vi "Get Sibling Classes of Actor.vi"(7 "Target":refnum<vi>, 8 "error in (no error)":errorcluster, 11 "Actor":refnum<vi>) -> (0 "error out":errorcluster, 1 "Sibling Classes":refnum<vi>[](array[refnum]))   [LabVIEW 2020, in "Message Maker.lvlib"]
uses:
  Message Maker.lvlib
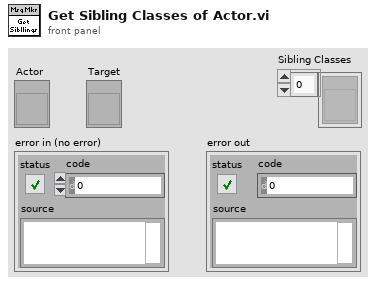
[diagram p1: front panel]
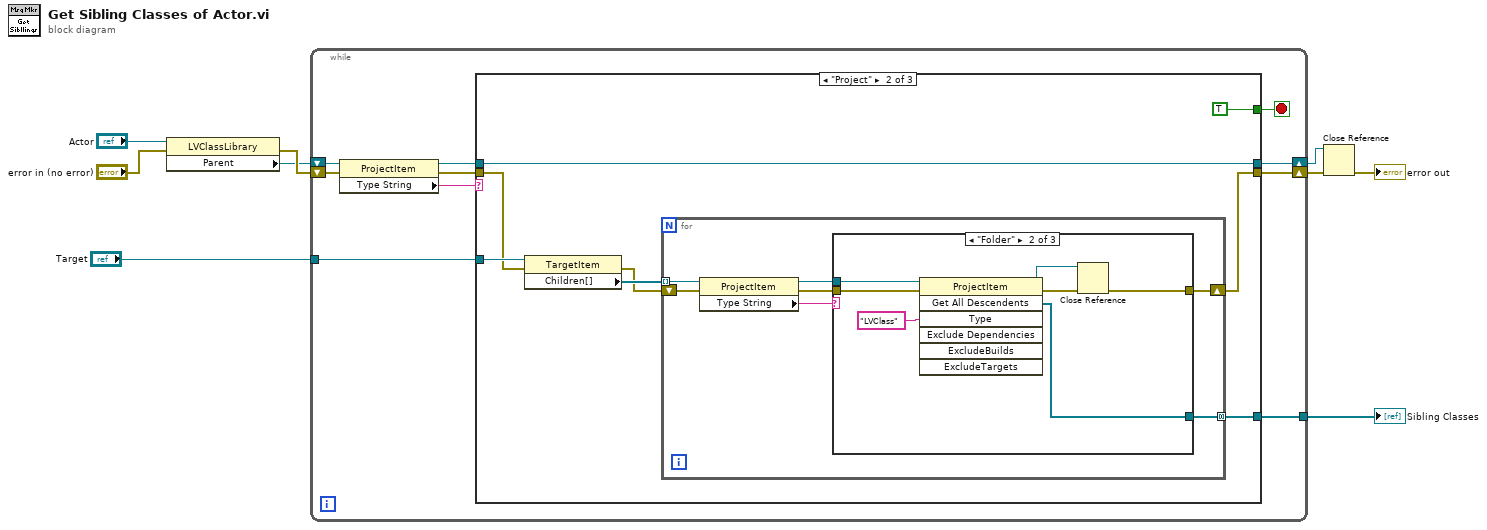
[diagram p0: block diagram]
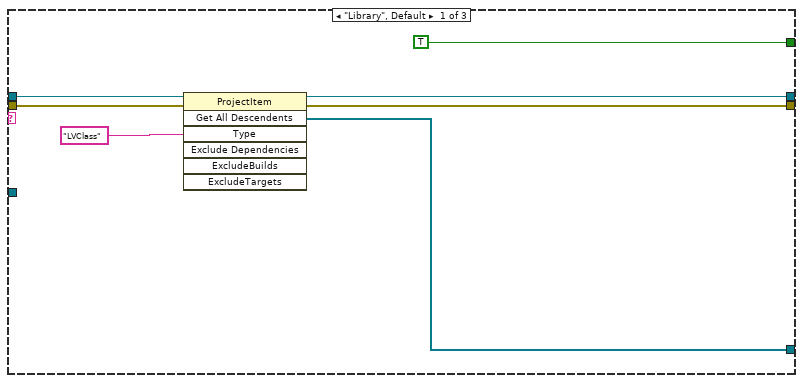
[diagram p2: hidden frame]
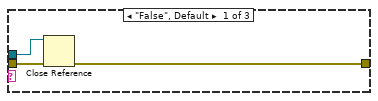
[diagram p3: hidden frame]
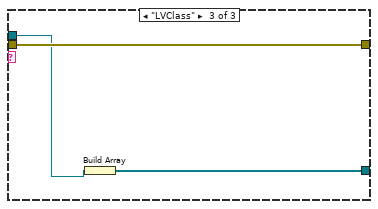
[diagram p4: hidden frame]
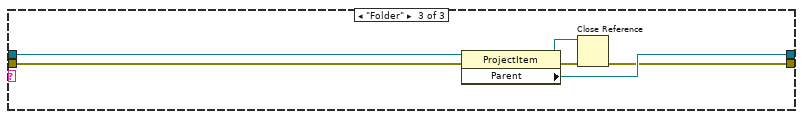
[diagram p5: hidden frame]
diagram:
  n1 = property class="LVClassLibrary"(reference="Actor", error in="error in (no error)") -> (error out=w8:errorcluster, "Parent"=w6:refnum<vi>)  [unwired: 1 out]
  n2 = while {
    shift-right: [w16] -> w4
    shift-left: w6 -> [w19]
    shift-right: [w13] -> w5
    shift-left: w8 -> [w15]
    tunnel: [w12] -> w1
    tunnel: "Target" -> [w10]
    stop <- w17 stop-if-true
    n3 = property class="ProjectItem"(reference=w19, error in=w15) -> (reference out=w11:refnum<vi>, error out=w14:errorcluster, "Type String"=w18:string)
    n4 = case shown="\"Project\"" w18 {
      tunnel: w11 -> [w25 w30 w60]
      tunnel: [w23 w30 w56] -> w16
      tunnel: [TRUE TRUE _] -> w17
      tunnel: w14 -> [w24 w31 w59]
      tunnel: [w22 w28 w55] -> w13
      tunnel: [w20 w27 _] -> w12
      tunnel: w10 -> [_ w32 _]
      frame "Library", Default {
        n5 = invoke class="ProjectItem" method="Get All Descendents"(reference=w25, error in=w24, "Type"="LVClass") -> (reference out=w23:refnum<vi>, error out=w22:errorcluster, "All Descendents"=w20:refnum<vi>[])  [unwired: 4 in, 4 out]
      }
      frame "Project" {
        n6 = property class="TargetItem"(reference=w32, error in=w31) -> (error out=w29:errorcluster, "Children[]"=w33:refnum<vi>[])  [unwired: 1 out]
        n7 = for {
          tunnel: w33 -> [w41] mode=indexing
          shift-right: [w35] -> w28
          shift-left: w29 -> [w36]
          tunnel: [w39] -> w27 mode=concatenating
          n8 = property class="ProjectItem"(reference=w41, error in=w36) -> (reference out=w38:refnum<vi>, error out=w37:errorcluster, "Type String"=w40:string)
          n9 = case shown="\"Folder\"" w40 {
            tunnel: [_ w45 w54] -> w39
            tunnel: w38 -> [w43 w50 w52]
            tunnel: w37 -> [w44 w47 w53]
            tunnel: [w42 w46 w53] -> w35
            frame "False", Default {
              n10 = Close Reference(reference=w43, error in (no error)=w44) -> (error out=w42:errorcluster)
            }
            frame "Folder" {
              n11 = invoke class="ProjectItem" method="Get All Descendents"(reference=w50, error in=w47, "Type"="LVClass") -> (reference out=w48:refnum<vi>, error out=w49:errorcluster, "All Descendents"=w45:refnum<vi>[])  [unwired: 4 in, 4 out]
              n12 = Close Reference(reference=w48, error in (no error)=w49) -> (error out=w46:errorcluster)
            }
            frame "LVClass" {
              n13 = Build Array(w52) -> (w54:refnum<vi>[])
            }
          }
        }
      }
      frame "Folder" {
        n14 = property class="ProjectItem"(reference=w60, error in=w59) -> (reference out=w57:refnum<vi>, error out=w58:errorcluster, "Parent"=w56:refnum<vi>)
        n15 = Close Reference(reference=w57, error in (no error)=w58) -> (error out=w55:errorcluster)
      }
    }
  }
  "Sibling Classes" <- w1
  n16 = Close Reference(reference=w4, error in (no error)=w5) -> (error out=→"error out":errorcluster)
